vi "monochromatorGetResponseSTR.vi"(8 "error in":errorcluster, 10 "command":string, 11 "monochromator":refnum<k24>) -> (0 "error out":errorcluster, 2 "response":string, 3 "reference out":refnum<k24>)   [LabVIEW 2009]
doc: "This VI accepts string command and returns response from the monochromator as INT\nBoth the command and monochromator vars are required\nIf connected error cluster contains error, command will not be sent and this VI will return NaV as response."
uses:
  C:/Users/anderson.chen/Desktop/Software Development/Cornerstone Series API (LV9)/Cornerstone DLL/Cornerstone.dll
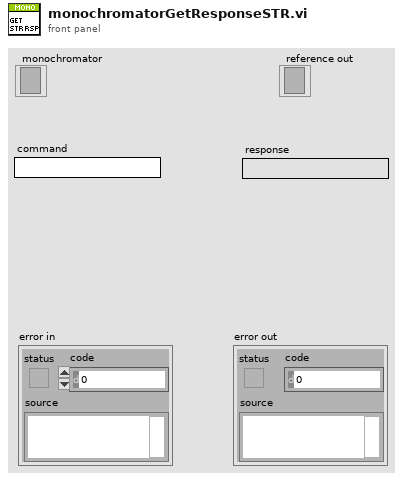
[diagram p1: front panel]
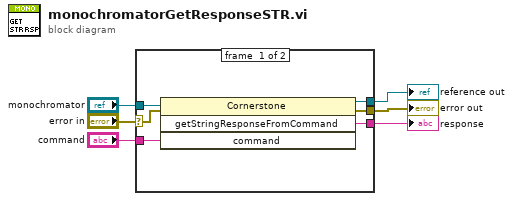
[diagram p0: block diagram]
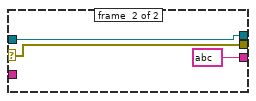
[diagram p2: hidden frame]
diagram:
  n1 = case shown="Error" "error in" {
    selector: "error in" -> [w7 w15]
    tunnel: "monochromator" -> [w12 w14]
    tunnel: "command" -> [w11 _]
    tunnel: [w10 string ? ("getStringResponseFromCommand")] -> w1
    tunnel: [w9 w14] -> w4
    tunnel: [w8 w15] -> w3
    frame #0 {
      n2 = invoke class="Cornerstone" method="getStringResponseFromCommand"(reference=w12, error in=w7, "command"=w11) -> (reference out=w9:refnum<k24>, error out=w8:errorcluster, "getStringResponseFromCommand"=w10:string)  [unwired: 1 in, 1 out]
    }
    frame #1 {
    }
  }
  "reference out" <- w4
  "error out" <- w3
  "response" <- w1
